vi "Reading Rokubi Serial.vi"() -> ()   [LabVIEW 2019]
uses:
  <vilib>/Instr/_visa.llb/VISA Configure Serial Port (Instr).vi
panel:
  out "Mz off":sgl
  out "My off":sgl
  out "Mx off":sgl
  out "Fz off":sgl
  out "Fy off":sgl
  out "Fx off":sgl
  in  "Calculate offset":bool
  out "Fx graph":sgl[](graph)
  out "Fy graph":sgl[](graph)
  out "Fz graph":sgl[](graph)
  out "Mx graph":sgl[](graph)
  out "My graph":sgl[](graph)
  out "Mz graph":sgl[](graph)
  out "Thermometer":sgl(slide) scale=0.0..50.0
  out "Temp (C)":sgl
  out "Mz (Nm)":sgl format="%#.2g"
  out "My (Nm)":sgl format="%#.2g"
  out "Mx (Nm)":sgl format="%#.2g"
  out "Fz (N)":sgl format="%#.2g"
  out "Fy (N)":sgl format="%#.2g"
  out "Fx (N)":sgl format="%#.2g"
  out "String 2":string
  out "Status":string
  in  "stop":bool
  out "String":string
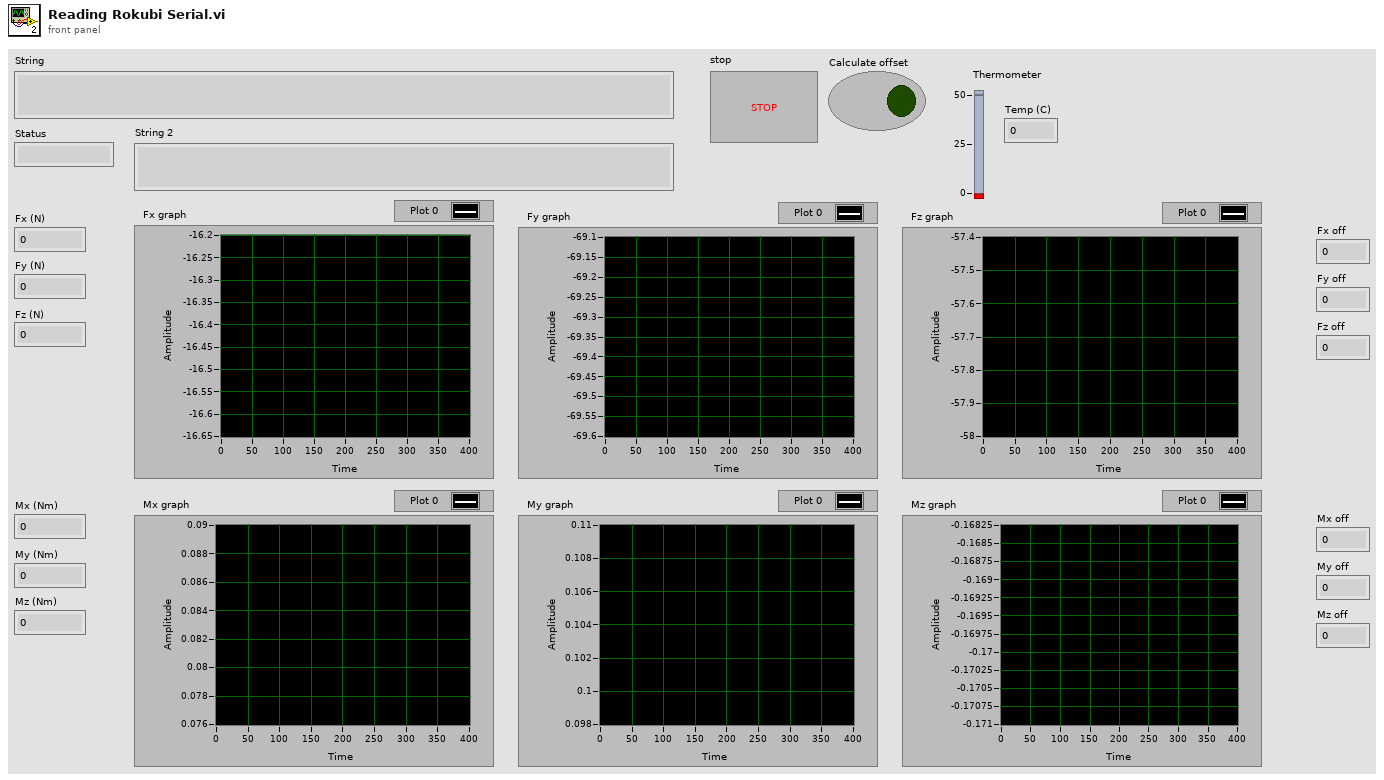
[diagram p1: front panel]
types:
  T1 = enum16{"big-endian, network order", "native, host order", "little-endian"}
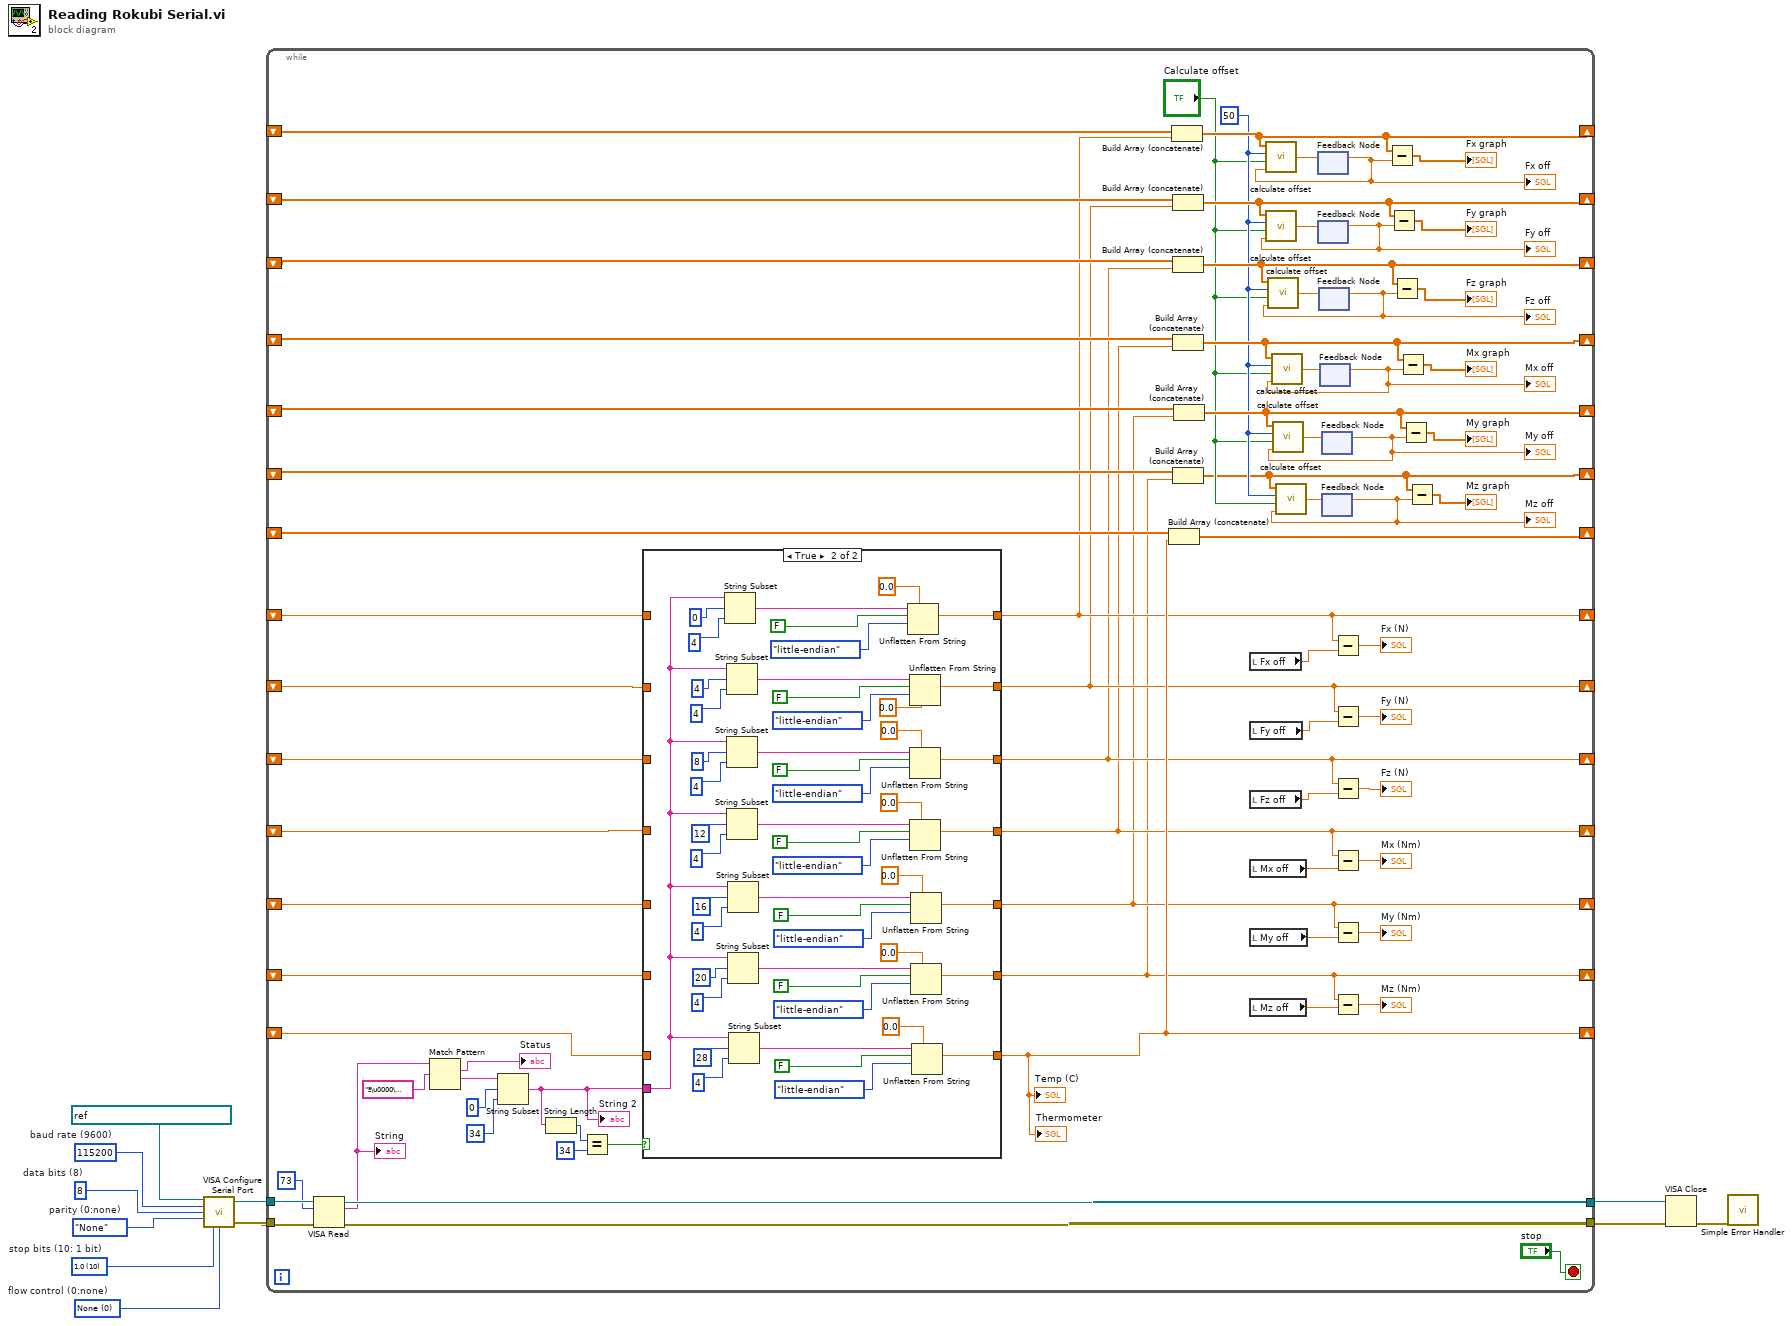
[diagram p0: block diagram]
diagram:
  w4 = u16 0 items=["None", "XON/XOFF", "RTS/CTS", "XON/XOFF & RTS/CTS", "DTR/DSR", "XON/XOFF & DTR/DSR"]  # flow control (0:none)
  w5 = u16 10 items=["1.0"=10, "1.5"=15, "2.0"=20]  # stop bits (10: 1 bit)
  w6 = enum16{"None", "Odd", "Even", "Mark", "Space"}."None"  # parity (0:none)
  w7 = u16 8  # data bits (8)
  w11 = u32 115200  # baud rate (9600)
  n1 = call-poly "VISA Configure Serial Port"("VISA resource name"=refnum<visa-resource-name> "visa://172.22.11.2/Rokubi", "baud rate (9600)"=w11, "data bits (8)"=w7, "parity (0:none)"=w6, "stop bits (10: 1 bit)"=w5, "flow control (0:none)"=w4) -> ("VISA resource name out"=w3:refnum<visa-resource-name>, "error out"=w2:errorcluster)  [unwired: 8 in]
  n2 = while {
    tunnel: [w86] -> w10
    tunnel: [w85] -> w9
    tunnel: w3 -> [w84]
    tunnel: w2 -> [w83]
    shift-right: [w30] -> _
    shift-left: _ -> [w72]
    shift-right: [w29] -> _
    shift-left: _ -> [w70]
    shift-right: [w28] -> _
    shift-left: _ -> [w69]
    shift-right: [w27] -> _
    shift-left: _ -> [w68]
    shift-right: [w26] -> _
    shift-left: _ -> [w67]
    shift-right: [w25] -> _
    shift-left: _ -> [w66]
    shift-right: [w62] -> _
    shift-left: _ -> [w65]
    shift-right: [w63] -> _
    shift-left: _ -> [w64]
    shift-right: [w39] -> _
    shift-left: _ -> [w42]
    shift-right: [w44] -> _
    shift-left: _ -> [w46]
    shift-right: [w48] -> _
    shift-left: _ -> [w49]
    shift-right: [w52] -> _
    shift-left: _ -> [w53]
    shift-right: [w56] -> _
    shift-left: _ -> [w57]
    shift-right: [w59] -> _
    shift-left: _ -> [w61]
    stop <- "stop" stop-if-true
    w41 = 50 ("avg of")
    n3 = VISA Read(VISA resource name=w84, byte count=u32 73, error in (no error)=w83) -> (VISA resource name out=w86:refnum<visa-resource-name>, read buffer=w79:string, error out=w85:errorcluster)  [unwired: 1 out]
    "String" <- w79
    n4 = Match Pattern(string=w79, regular expression="ª\u0000\u0000" ("y")) -> (match substring=→"Status":string, after substring=w77:string)  [unwired: 1 in, 2 out]
    n5 = String Subset(string=w77, offset (0)=0, length (rest)=34 ("length (rest)")) -> (substring=w71:string)
    "String 2" <- w71
    n6 = String Length(string=w71) -> (length=w74:i32)
    n7 = Equal?(x=w74, y=34) -> (x = y?=w75:bool)
    n8 = case shown="True" w75 {
      tunnel: w71 -> [_ w101]
      tunnel: [w88 w138] -> w30
      tunnel: w72 -> [w88 _]
      tunnel: [w94 w100] -> w29
      tunnel: [w93 w99] -> w28
      tunnel: [w92 w98] -> w27
      tunnel: [w91 w97] -> w26
      tunnel: [w90 w96] -> w25
      tunnel: [w89 w95] -> w62
      tunnel: w70 -> [w94 _]
      tunnel: w69 -> [w93 _]
      tunnel: w68 -> [w92 _]
      tunnel: w67 -> [w91 _]
      tunnel: w66 -> [w90 _]
      tunnel: w65 -> [w89 _]
      frame False {
      }
      frame True {
        n9 = String Subset(string=w101, offset (0)=0, length (rest)=4) -> (substring=w139:string)
        n10 = String Subset(string=w101, offset (0)=4, length (rest)=4) -> (substring=w132:string)
        n11 = String Subset(string=w101, offset (0)=8, length (rest)=4) -> (substring=w126:string)
        n12 = String Subset(string=w101, offset (0)=12, length (rest)=4) -> (substring=w120:string)
        n13 = String Subset(string=w101, offset (0)=16, length (rest)=4) -> (substring=w114:string)
        n14 = String Subset(string=w101, offset (0)=20, length (rest)=4) -> (substring=w108:string)
        n15 = String Subset(string=w101, offset (0)=28, length (rest)=4) -> (substring=w102:string)
        n16 = Unflatten From String(type=sgl 0.0, binary string=w139, data includes array or string size? (T)=FALSE, byte order (0:big-endian, network order)=T1."little-endian") -> (value=w138:sgl)  [unwired: 1 in, 2 out]
        n17 = Unflatten From String(type=sgl 0.0, binary string=w132, data includes array or string size? (T)=FALSE, byte order (0:big-endian, network order)=T1."little-endian") -> (value=w100:sgl)  [unwired: 1 in, 2 out]
        n18 = Unflatten From String(type=sgl 0.0, binary string=w126, data includes array or string size? (T)=FALSE, byte order (0:big-endian, network order)=T1."little-endian") -> (value=w99:sgl)  [unwired: 1 in, 2 out]
        n19 = Unflatten From String(type=sgl 0.0, binary string=w120, data includes array or string size? (T)=FALSE, byte order (0:big-endian, network order)=T1."little-endian") -> (value=w98:sgl)  [unwired: 1 in, 2 out]
        n20 = Unflatten From String(type=sgl 0.0, binary string=w114, data includes array or string size? (T)=FALSE, byte order (0:big-endian, network order)=T1."little-endian") -> (value=w97:sgl)  [unwired: 1 in, 2 out]
        n21 = Unflatten From String(type=sgl 0.0, binary string=w108, data includes array or string size? (T)=FALSE, byte order (0:big-endian, network order)=T1."little-endian") -> (value=w96:sgl)  [unwired: 1 in, 2 out]
        n22 = Unflatten From String(type=sgl 0.0, binary string=w102, data includes array or string size? (T)=FALSE, byte order (0:big-endian, network order)=T1."little-endian") -> (value=w95:sgl)  [unwired: 1 in, 2 out]
      }
    }
    "Temp (C)" <- w62
    "Thermometer" <- w62
    n23 = Build Array (concatenate)(w64, w62) -> (w63:sgl[])
    n24 = Build Array (concatenate)(w61, w30) -> (w59:sgl[])
    n25 = Build Array (concatenate)(w57, w29) -> (w56:sgl[])
    n26 = Build Array (concatenate)(w53, w28) -> (w52:sgl[])
    n27 = Build Array (concatenate)(w49, w27) -> (w48:sgl[])
    n28 = Build Array (concatenate)(w42, w25) -> (w39:sgl[])
    n29 = Build Array (concatenate)(w46, w26) -> (w44:sgl[])
    n30 = local read "Fx off"() -> (w17:sgl)
    n31 = local read "Fy off"() -> (w16:sgl)
    n32 = local read "Fz off"() -> (w15:sgl)
    n33 = local read "Mx off"() -> (w14:sgl)
    n34 = local read "My off"() -> (w13:sgl)
    n35 = local read "Mz off"() -> (w12:sgl)
    n36 = feedback #1() -> (w23:sgl)  [unwired: 1 in]
    "Fx off" <- w23
    n37 = call "calculate offset.vi"("outpin in"=w23, "Calculate offset"="Calculate offset", "avg of"=w41, "numeric array"=w59) -> ("Offset"=w58:sgl)
    n38 = feedback-in #1(w58) -> ()
    n39 = feedback #2() -> (w22:sgl)  [unwired: 1 in]
    "Fy off" <- w22
    n40 = call "calculate offset.vi"("outpin in"=w22, "Calculate offset"="Calculate offset", "avg of"=w41, "numeric array"=w56) -> ("Offset"=w54:sgl)
    n41 = feedback-in #2(w54) -> ()
    n42 = feedback #3() -> (w21:sgl)  [unwired: 1 in]
    "Fz off" <- w21
    n43 = call "calculate offset.vi"("outpin in"=w21, "Calculate offset"="Calculate offset", "avg of"=w41, "numeric array"=w52) -> ("Offset"=w50:sgl)
    n44 = feedback-in #3(w50) -> ()
    n45 = feedback #4() -> (w20:sgl)  [unwired: 1 in]
    "Mx off" <- w20
    n46 = call "calculate offset.vi"("outpin in"=w20, "Calculate offset"="Calculate offset", "avg of"=w41, "numeric array"=w48) -> ("Offset"=w47:sgl)
    n47 = feedback-in #4(w47) -> ()
    n48 = feedback #5() -> (w19:sgl)  [unwired: 1 in]
    "My off" <- w19
    n49 = call "calculate offset.vi"("outpin in"=w19, "Calculate offset"="Calculate offset", "avg of"=w41, "numeric array"=w44) -> ("Offset"=w43:sgl)
    n50 = feedback-in #5(w43) -> ()
    n51 = feedback #6() -> (w18:sgl)  [unwired: 1 in]
    "Mz off" <- w18
    n52 = call "calculate offset.vi"("outpin in"=w18, "Calculate offset"="Calculate offset", "avg of"=w41, "numeric array"=w39) -> ("Offset"=w37:sgl)
    n53 = feedback-in #6(w37) -> ()
    n54 = Subtract(x=w30, y=w17) -> (x-y=→"Fx (N)":sgl)
    n55 = Subtract(x=w29, y=w16) -> (x-y=→"Fy (N)":sgl)
    n56 = Subtract(x=w28, y=w15) -> (x-y=→"Fz (N)":sgl)
    n57 = Subtract(x=w27, y=w14) -> (x-y=→"Mx (Nm)":sgl)
    n58 = Subtract(x=w26, y=w13) -> (x-y=→"My (Nm)":sgl)
    n59 = Subtract(x=w25, y=w12) -> (x-y=→"Mz (Nm)":sgl)
    n60 = Subtract(x=w59, y=w23) -> (x-y=→"Fx graph":sgl[])
    n61 = Subtract(x=w56, y=w22) -> (x-y=→"Fy graph":sgl[])
    n62 = Subtract(x=w52, y=w21) -> (x-y=→"Fz graph":sgl[])
    n63 = Subtract(x=w48, y=w20) -> (x-y=→"Mx graph":sgl[])
    n64 = Subtract(x=w44, y=w19) -> (x-y=→"My graph":sgl[])
    n65 = Subtract(x=w39, y=w18) -> (x-y=→"Mz graph":sgl[])
  }
  n66 = VISA Close(VISA resource name=w10, error in (no error)=w9) -> (error out=w8:errorcluster)
  n67 = call <vilib>:"Simple Error Handler.vi"("error in (no error)"=w8) -> ()  [unwired: 1 in, 8 out]
